vi "Initialise.vi"(8 "error in (no error)":errorcluster, 10 "Message in":refnum<class "InitialiseMessage.lvclass">, 11 "DAQMH121119OrcaFlash in":refnum<class "DAQOrcaFlash.lvclass">) -> (0 "error out":errorcluster, 3 "DAQMH121119OrcaFlash out":refnum<class "DAQOrcaFlash.lvclass">)   [LabVIEW 2012, in "DAQOrcaFlash.lvclass"]
doc: "This member function is called when the statemachine in the run.vi receives an 'initialise' message. It mainly initialises the RabbitMQ connectivity. \n\nOverride this member function in your derived class to initialise hardware or software resources (but don't forget to call the parent method). If your component owns subcomponents, they count as resources, so you have to initialise them by calling their own initialise functions."
uses:
  DAQOrcaFlash.lvclass
  <vilib>/Distrio/Murmex/InitialiseMessage/InitialiseMessage.lvclass
  <vilib>/Distrio/Murmex/Murmex/Murmex.lvclass
  <vilib>/Distrio/Murmex/TerminateMessage/TerminateMessage.lvclass
  <vilib>/Distrio/Murmex/UpdateMessage/UpdateMessage.lvclass
  imaging_mode.ctl
  DAQOrcaFlash.lvclass/DAQOrcaFlash.ctl
  <vilib>/Distrio/Murmex/GenericMessage/GenericMessage.lvclass
  <vilib>/Distrio/Murmex/Message/Add or replace parameter.vi
panel:
  # "This method is called when the INTIALISE\ntrigger is sent. \n\nOverride this method when your component needs to\nrespond to this trigger. \n\nCall parent for proper implementation"
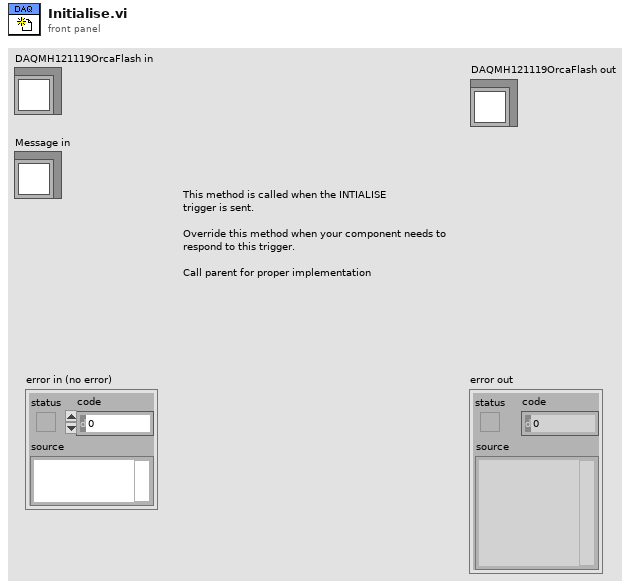
[diagram p1: front panel]
types:
  T1 = typedef "DAQOrcaFlash.lvclass/imaging_mode.ctl" = enum16{"focus mode", "single sweep"}
  T2 = cluster{"Mode":u32, "Polarity":u32, "Period":dbl, "Delay":dbl}
  T3 = typedef "Image Type" = u32
  T4 = typedef "IMAQ Image.ctl" = refnum<image>
  T5 = cluster{"height":u32, "width":u32, "datatype":u32}
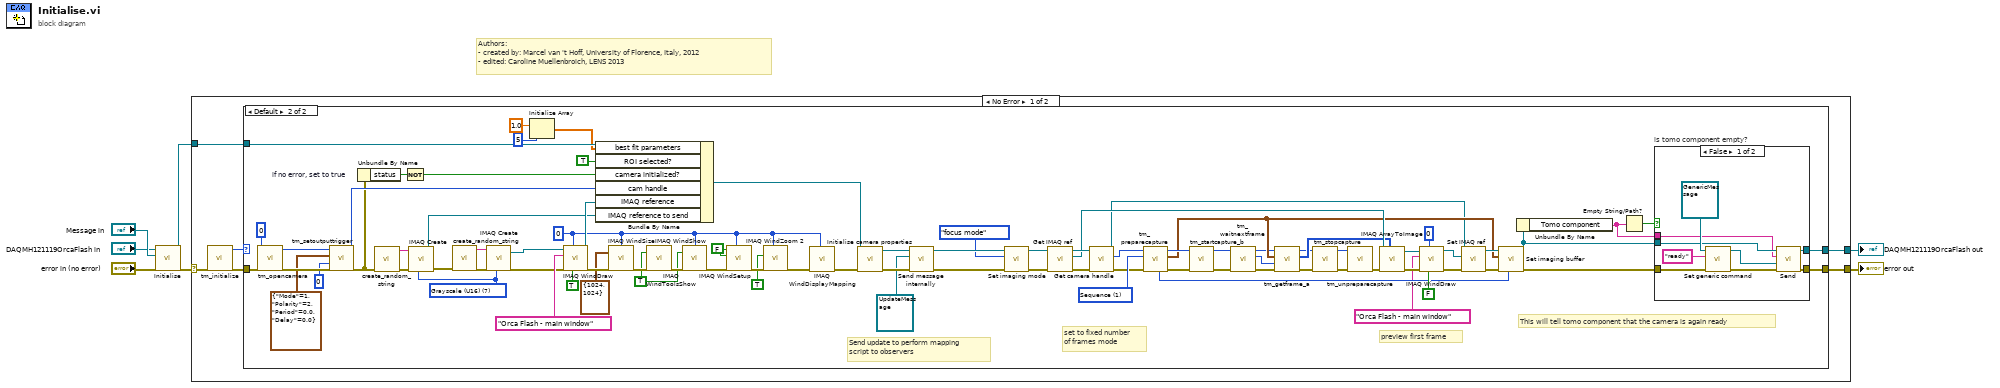
[diagram p0: block diagram]
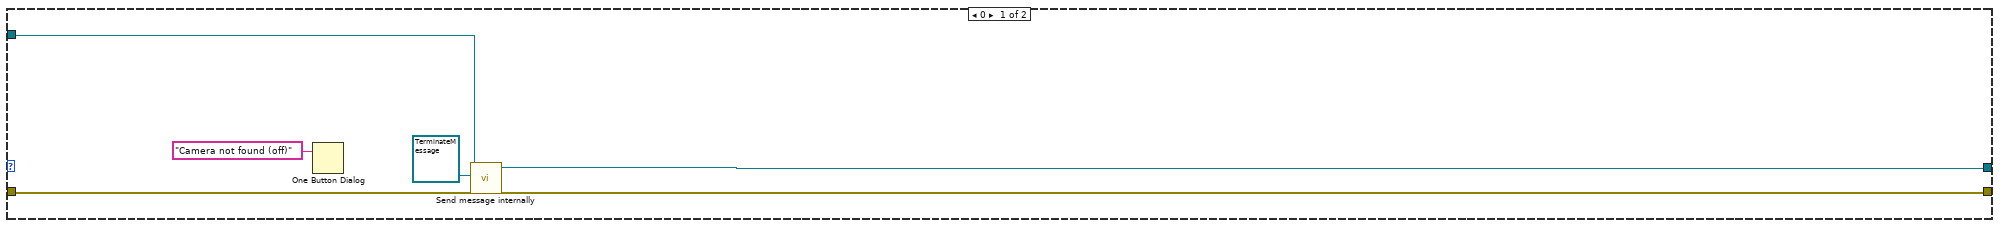
[diagram p2: hidden frame]
diagram:
  # "Authors: \n- created by: Marcel van 't Hoff, University of Florence, Italy, 2012\n- edited: Caroline Muellenbroich, LENS 2013"
  n1 = call-parent "Initialise.vi"("error in (no error)"="error in (no error)", "Message in"="Message in", "Murmex in"="DAQMH121119OrcaFlash in") -> ("error out"=w4:errorcluster, "Murmex out"=w3:refnum<class "DAQOrcaFlash.lvclass">)  [unwired: 7 in]
  n2 = case shown="No Error" w4 {
    selector: w4 -> [w12 w116]
    tunnel: w3 -> [w11 w117]
    tunnel: [w10 w117] -> w2
    tunnel: [w9 w116] -> w1
    frame No Error {
      n3 = call <userlib>:"tm_initialize.vi"("error in (no error)"=w12) -> ("error out"=w13:errorcluster, "Number Of Cameras"=w8:u32)  [unwired: 7 in, 2 out]
      n4 = case shown="Default" w8 {
        tunnel: w13 -> [w19 w104]
        tunnel: w11 -> [w17 w100]
        tunnel: [w16 w26] -> w10
        tunnel: [w18 w28] -> w9
        frame 0 {
          n5 = One Button Dialog(message="Camera not found (off)") -> ()  [unwired: 1 in, 1 out]
          n6 = call <vilib>:"Send message internally.vi"("error in (no error)"=w19, "Message"=refnum<class "TerminateMessage.lvclass"> refnum ("TerminateMessage"), "Murmex in"=w17) -> ("error out"=w18:errorcluster, "Murmex out"=w16:refnum<class "DAQOrcaFlash.lvclass">)  [unwired: 7 in]
        }
        frame Default {
          w58 = 1 items=["Snap", "Sequence"] ("Capture mode")
          w88 = FALSE ("Window can grow? (Yes)")
          w66 = 0 ("Window Number (0...15)")
          w90 = TRUE ("Hide/Show (Show)")
          w77 = T3 7 items=["Grayscale (U8)", "Grayscale (I16)", "Grayscale (SGL)", "Complex (CSG)", "RGB (U32)", "HSL (U32)", "RGB (U64)", "Grayscale (U16)"] ("Image Type")
          # "This will tell tomo component that the camera is again ready"
          # "preview first frame"
          # "set to fixed number\nof frames mode"
          # "Send update to perform mapping\nscript to observers"
          n7 = call <userlib>:"tm_opencamera.vi"("error in (no error)"=w104, "Camera Index"=u32 0) -> ("error out"=w84:errorcluster, "Handle out"=w85:u32)  [unwired: 7 in, 1 out]
          n8 = call <userlib>:"tm_setoutputtrigger.vi"("error in (no error)"=w84, "Index"=0, "Parameters"=T2 {"Mode"=1, "Polarity"=2, "Period"=0.0, "Delay"=0.0}, "Handle in"=w85) -> ("error out"=w71:errorcluster, "Handle out"=w81:u32)  [unwired: 6 in]
          n9 = Unbundle By Name "if no error, set to true"(w71) -> ("status"=w70:bool)
          n10 = call "create_random_string.vi"("error in (no error)"=w71) -> ("error out"=w78:errorcluster, "random string"=w76:string)  [unwired: 9 in]
          n11 = Not(x=w70) -> (.not. x?=w69:bool)
          n12 = call "IMAQ Create"("Image Name"=w76, "Image Type"=w77, "error in (no error)"=w78) -> ("New Image"=w75:T4, "error out"=w79:errorcluster)  [unwired: 2 in]
          n13 = call "create_random_string.vi"("error in (no error)"=w79) -> ("error out"=w102:errorcluster, "random string"=w101:string)  [unwired: 9 in]
          n14 = call "IMAQ Create"("Image Name"=w101, "Image Type"=w77, "error in (no error)"=w102) -> ("New Image"=w97:T4, "error out"=w94:errorcluster)  [unwired: 2 in]
          n15 = Initialize Array(1.0 ("element"), 5 ("dimension size")) -> (w20:dbl[])
          n16 = call "IMAQ WindDraw"("Resize to Image Size? (Y)"=TRUE, "Window Number (0...15)"=w66, "error in (no error)"=w94, "Title"="Orca Flash - main window", "Image"=w97) -> ("error out"=w93:errorcluster, "Image Out (duplicate)"=w98:T4)  [unwired: 5 in]
          n17 = Bundle By Name(cluster=w100, "best fit parameters"=w20, "ROI selected?"=TRUE ("Runtime cluster.ROI selected?"), "camera initialized?"=w69, "cam handle"=w81, "IMAQ reference"=w98, "IMAQ reference to send"=w75) -> (w80:refnum<class "DAQOrcaFlash.lvclass">)
          n18 = call "IMAQ WindSize"("error in (no error)"=w93, "Width & Height"=cluster{"Width":i32, "Height":i32} {"Width"=1024, "Height"=1024}, "Window Number"=w66) -> ("error out"=w92:errorcluster)  [unwired: 3 in, 2 out]
          n19 = call "IMAQ WindToolsShow"("Hide/Show (Show)"=w90, "error in (no error)"=w92) -> ("error out"=w99:errorcluster)  [unwired: 3 in, 1 out]
          n20 = call "IMAQ WindShow"("error in (no error)"=w99, "Hide/Show (Show)"=w90, "Window Number (0...15)"=w66) -> ("error out"=w89:errorcluster)  [unwired: 3 in, 2 out]
          n21 = call "IMAQ WindSetup"("Window Number (0...15)"=w66, "error in (no error)"=w89, "Window can close? (Yes)"=w88, "Window can grow? (Yes)"=w88) -> ("error out"=w87:errorcluster)  [unwired: 7 in]
          n22 = call "IMAQ WindZoom 2"("Window Number (0...15)"=w66, "error in (no error)"=w87, "Zoom to Fit? (False)"=TRUE) -> ("error out"=w68:errorcluster)  [unwired: 5 in, 3 out]
          n23 = call "IMAQ WindDisplayMapping"("Window Number (0...15)"=w66, "error in (no error)"=w68) -> ("error out"=w67:errorcluster)  [unwired: 8 in, 1 out]
          n24 = call-dynamic "Initialise camera properties.vi"("error in (no error)"=w67, "DAQOrcaFlash in"=w80) -> ("error out"=w74:errorcluster, "DAQOrcaFlash out"=w73:refnum<class "DAQOrcaFlash.lvclass">)  [unwired: 8 in]
          n25 = call <vilib>:"Send message internally.vi"("error in (no error)"=w74, "Message"=refnum<class "UpdateMessage.lvclass"> refnum ("Distrio Murmex 1.0:UpdateMessage"), "Murmex in"=w73) -> ("error out"=w32:errorcluster, "Murmex out"=w30:refnum<class "DAQOrcaFlash.lvclass">)  [unwired: 7 in]
          n26 = call "Set imaging mode.vi"("error in (no error)"=w32, "imaging mode"=imaging_mode."focus mode", "DAQMH121119OrcaFlash in"=w30) -> ("error out"=w33:errorcluster, "DAQMH121119OrcaFlash out"=w31:refnum<class "DAQOrcaFlash.lvclass">)  [unwired: 7 in]
          n27 = call "Get IMAQ ref.vi"("error in (no error)"=w33, "DAQMH121119OrcaFlash in"=w31) -> ("error out"=w64:errorcluster, "IMAQ reference"=w53:T4, "DAQMH121119OrcaFlash out"=w65:refnum<class "DAQOrcaFlash.lvclass">)  [unwired: 7 in]
          n28 = call "Get camera handle.vi"("error in (no error)"=w64, "DAQMH121119OrcaFlash in"=w65) -> ("error out"=w43:errorcluster, "cam handle"=w44:u32, "DAQMH121119OrcaFlash out"=w47:refnum<class "DAQOrcaFlash.lvclass">)  [unwired: 7 in]
          n29 = call <userlib>:"tm_preparecapture.vi"("error in (no error)"=w43, "Capture mode"=w58, "Handle in"=w44) -> ("error out"=w59:errorcluster, "Buffer Info"=w51:T5, "Handle out"=w57:u32, "Image type"=w50:u32)  [unwired: 5 in]
          n30 = call <userlib>:"tm_startcapture_b.vi"("error in (no error)"=w59, "Handle in"=w57) -> ("error out"=w56:errorcluster, "Handle out"=w34:u32)  [unwired: 8 in]
          n31 = call <userlib>:"tm_waitnextframe.vi"("error in (no error)"=w56, "Handle in"=w34) -> ("error out"=w42:errorcluster, "Frame Index"=w55:i32, "Handle out"=w41:u32)  [unwired: 6 in, 1 out]
          n32 = call <userlib>:"tm_getframe_a.vi"("error in (no error)"=w42, "Frame Index"=w55, "Buffer Info"=w51, "Handle in"=w41) -> ("error out"=w37:errorcluster, "Data 16"=w49:u16[][], "Handle out"=w40:u32)  [unwired: 3 in, 2 out]
          n33 = call <userlib>:"tm_stopcapture.vi"("error in (no error)"=w37, "Handle in"=w40) -> ("error out"=w38:errorcluster, "Handle out"=w39:u32)  [unwired: 8 in]
          n34 = call <userlib>:"tm_unpreparecapture.vi"("error in (no error)"=w38, "Handle in"=w39) -> ("error out"=w36:errorcluster)  [unwired: 8 in, 1 out]
          n35 = call "IMAQ ArrayToImage"("Image Pixels (U16)"=w49, "error in (no error)"=w36, "Image"=w53) -> ("error out"=w54:errorcluster, "Image Out"=w52:T4)  [unwired: 7 in]
          n36 = call "IMAQ WindDraw"("Resize to Image Size? (Y)"=FALSE, "Window Number (0...15)"=0, "error in (no error)"=w54, "Title"="Orca Flash - main window", "Image"=w52) -> ("error out"=w61:errorcluster, "Image Out (duplicate)"=w48:T4)  [unwired: 5 in]
          n37 = call "Set IMAQ ref.vi"("error in (no error)"=w61, "IMAQ reference"=w48, "DAQMH121119OrcaFlash in"=w47) -> ("error out"=w62:errorcluster, "DAQMH121119OrcaFlash out"=w63:refnum<class "DAQOrcaFlash.lvclass">)  [unwired: 7 in]
          n38 = call "Set imaging buffer.vi"("Image type"=w50, "error in (no error)"=w62, "Buffer"=w51, "DAQMH121119OrcaFlash in"=w63) -> ("error out"=w35:errorcluster, "DAQMH121119OrcaFlash out"=w27:refnum<class "DAQOrcaFlash.lvclass">)  [unwired: 6 in]
          n39 = Unbundle By Name(w27) -> ("Tomo component"=w24:string)
          n40 = Empty String/Path?(string/path=w24) -> (empty?=w25:bool)
          n41 = case "is tomo component empty?" shown="False" w25 {
            tunnel: w35 -> [w113 w114]
            tunnel: [w111 w114] -> w28
            tunnel: w27 -> [w107 w115]
            tunnel: [w106 w115] -> w26
            tunnel: w24 -> [w105 _]
            frame False {
              n42 = call <vilib>:"Set generic command.vi"("error in (no error)"=w113, "generic command"="ready", "GenericMessage in"=refnum<class "GenericMessage.lvclass"> refnum ("Distrio Murmex 1.5:GenericMessage")) -> ("error out"=w112:errorcluster, "GenericMessage out"=w108:refnum<class "GenericMessage.lvclass">)  [unwired: 7 in]
              n43 = call <vilib>:"Send.vi"("error in (no error)"=w112, "Message"=w108, "recipient"=w105, "Murmex in"=w107) -> ("error out"=w111:errorcluster, "Murmex out"=w106:refnum<class "DAQOrcaFlash.lvclass">)  [unwired: 6 in]
            }
            frame True {
            }
          }
        }
      }
    }
    frame Error {
    }
  }
  "error out" <- w1
  "DAQMH121119OrcaFlash out" <- w2
